vi "InitAction.vi"(6 "InstrumentName":string, 7 "VisaRes":refnum<visa-resource-name>="COM1", 8 "error in (no error)":errorcluster caption="entrée d'erreur (pas d'erreur)", 9 "FirstClassInst":bool, 10 "Function":string, 11 "OR77200 In":refnum<class "OR77200.lvclass"> caption="DNL_LabVIEW Object in") -> (0 "error out":errorcluster caption="sortie d'erreur", 3 "OR77200 Out":refnum<class "OR77200.lvclass"> caption="DNL_LabVIEW Object out")   [LabVIEW 2019, in "OR77200.lvclass"]
uses:
  OR77200.lvclass
  C:/Programmes Labview/LabScanV1A/DevicesClass/BaseDevice/BaseDevice.lvclass
  OR77200_Func.ctl
panel:
  in  "OR77200_Func":T1
  out "VisaRes":refnum<visa-resource-name>
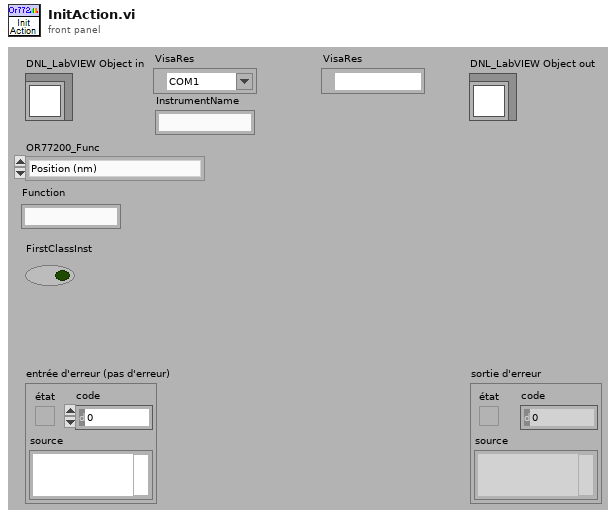
[diagram p1: front panel]
types:
  T1 = typedef "OR77200.lvclass/OR77200_Func.ctl" = enum16{"Position (nm)"}
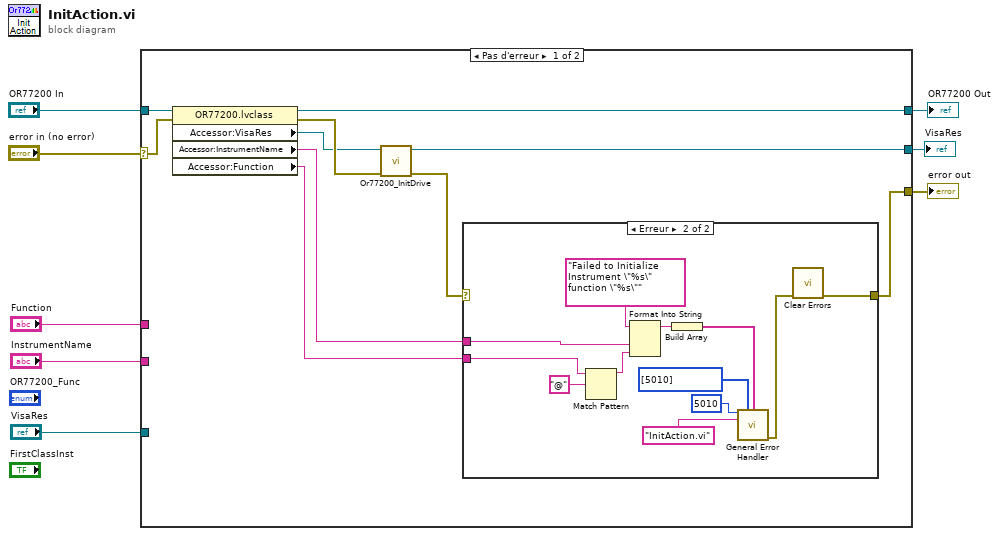
[diagram p0: block diagram]
diagram:
  n1 = case shown="Pas d'erreur" "error in (no error)" {
    selector: "error in (no error)" -> [w14 w33]
    tunnel: [w12 w33] -> w7
    tunnel: "OR77200 In" -> [w17 w32]
    tunnel: [w16 w32] -> w5
    tunnel: [w18 _] -> w4
    tunnel: "Function" -> [_ _]
    tunnel: "VisaRes" -> [_ _]
    tunnel: "InstrumentName" -> [_ _]
    frame No Error {
      n2 = property class="OR77200.lvclass"(reference=w17, error in=w14) -> (reference out=w16:refnum<class "OR77200.lvclass">, error out=w15:errorcluster, "Accessor:VisaRes"=w11:refnum<visa-resource-name>, "Accessor:InstrumentName"=w10:string, "Accessor:Function"=w9:string)
      n3 = call <userlib>:"Or77200_InitDrive.vi"("error In"=w15, "Port"=w11) -> ("sortie d'erreur"=w13:errorcluster, "Port Out"=w18:refnum<visa-resource-name>)  [unwired: 8 in]
      n4 = case shown="Erreur" w13 {
        selector: w13 -> [w19 _]
        tunnel: [w19 w20] -> w12
        tunnel: w10 -> [_ w23]
        tunnel: w9 -> [_ w22]
        frame No Error {
        }
        frame Error {
          n5 = Match Pattern(string=w22, regular expression="@" ("chaîne")) -> (before substring=w31:string)  [unwired: 1 in, 3 out]
          n6 = Format Into String(format string="Failed to Initialize Instrument \"%s\" function \"%s\"" ("[error source] (\" \")"), w23, w31) -> (resulting string=w26:string)  [unwired: 2 in, 1 out]
          n7 = Build Array(w26) -> (w25:string[])
          n8 = call <vilib>:"General Error Handler.vi"("[error code] (0)"=5010, "[user-defined codes]"=i32[] [5010], "[user-defined descriptions]"=w25, "[error source] (\" \")"="InitAction.vi" ("[error source] (\" \")")) -> ("error out"=w21:errorcluster)  [unwired: 7 in, 4 out]
          n9 = call <vilib>:"Clear Errors.vi"("error in (no error)"=w21) -> ("error out"=w20:errorcluster)  [unwired: 5 in, 1 out]
        }
      }
    }
    frame Error {
    }
  }
  "error out" <- w7
  "OR77200 Out" <- w5
  "VisaRes" <- w4
